vi "KlingerV2 GetStatus.vi"(4 "error in":errorcluster, 7 "VISA Rsrc":refnum<visa-resource-name>="SR530") -> (0 "error out":errorcluster, 1 "Message Cont":string caption="Message de statut", 2 "Statut":bool, 3 "Message D'erreur":string)   [LabVIEW 2019]
doc: "Ce VI effectue une lecture du message de statut du contrôlleur. Celui-ci indique entre autres, si les axes sont en mouvement, la positions de chaque axe, et l'état des interrupteurs de fin de course. De plus, si une erreur c'est produite (ex: commande invalide), il retourrne un code d'erreur avec une brève description. Dans ce dernier cas, le VI rapporte le message d'erreur au VI \"Klinger ErrorHandler\"."
uses:
  <vilib>/Utility/error.llb/DialogType.ctl
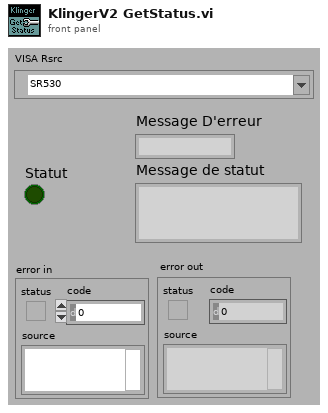
[diagram p1: front panel]
types:
  T1 = enum16{"Lit", "Fin", "Verif erreur", "fixe options", "commande ?"}
  T2 = typedef "DialogType.ctl" = u16
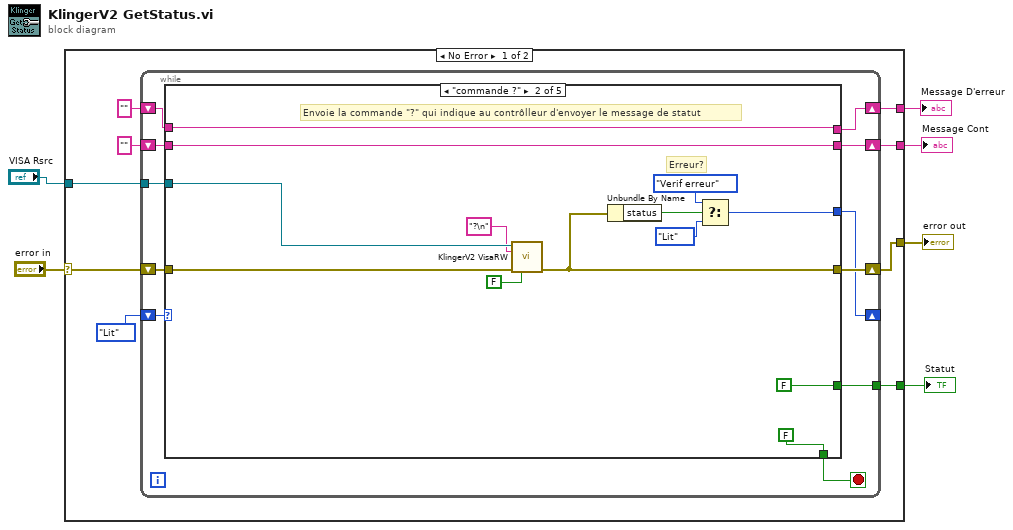
[diagram p0: block diagram]
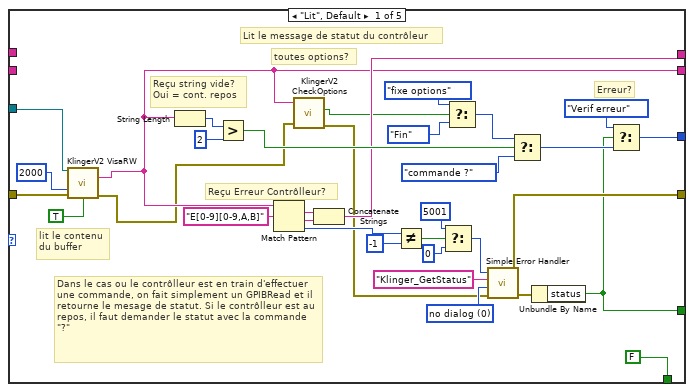
[diagram p2: hidden frame]
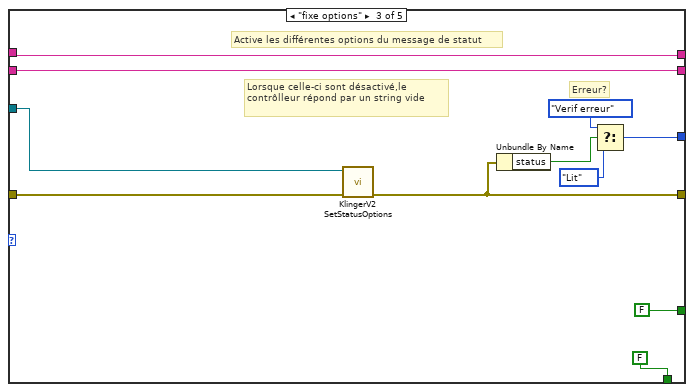
[diagram p3: hidden frame]
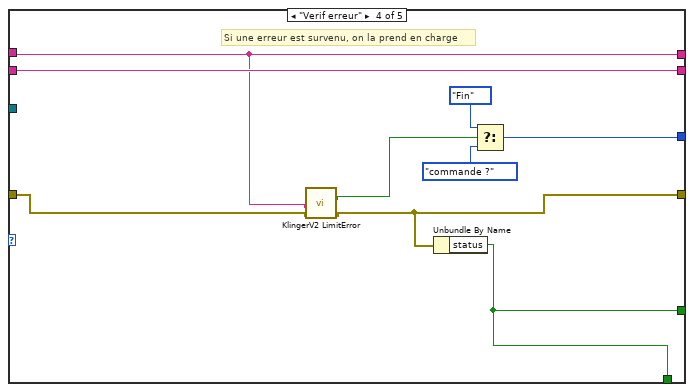
[diagram p4: hidden frame]
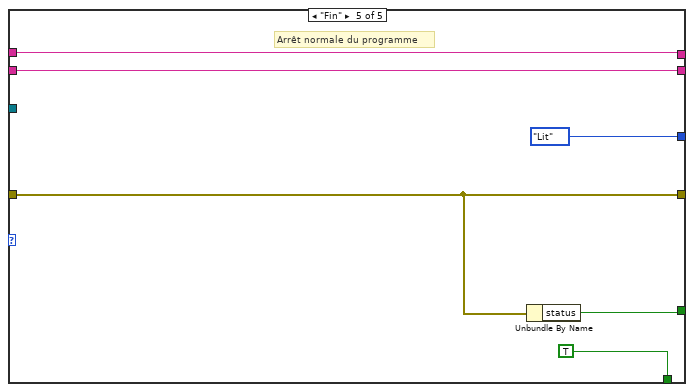
[diagram p5: hidden frame]
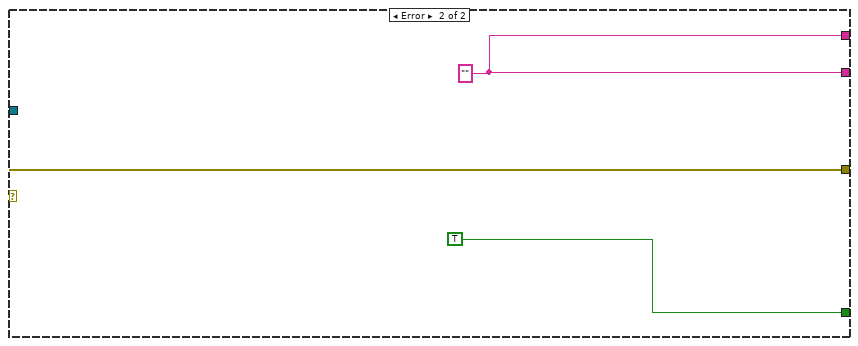
[diagram p6: hidden frame]
diagram:
  n1 = case shown="No Error" "error in" {
    selector: "error in" -> [w15 w101]
    tunnel: [w10 w99] -> w6
    tunnel: [w9 w101] -> w5
    tunnel: [w11 TRUE] -> w4
    tunnel: "VISA Rsrc" -> [w13 _]
    tunnel: [w14 w99] -> w2
    frame No Error {
      n2 = while {
        tunnel: w13 -> [w25]
        tunnel: [w21] -> w11
        shift-right: [w20] -> _
        shift-left: T1."Lit" -> [w24]
        shift-right: [w23] -> w9
        shift-left: w15 -> [w26]
        shift-right: [w22] -> w14
        shift-left: "" ("data") -> [w18]
        shift-right: [w16] -> w10
        shift-left: "" -> [w17]
        stop <- w19 stop-if-true
        n3 = case shown="\"commande ?\"" w24 {
          tunnel: w26 -> [w32 w62 w74 w85 w97]
          tunnel: [w31 w70 w82 w91 w95] -> w22
          tunnel: w25 -> [w30 w64 w75 _ _]
          tunnel: [w40 w61 w73 w86 w97] -> w23
          tunnel: [w39 FALSE FALSE ("status") w88 w98] -> w21
          tunnel: [w43 w65 w76 w92 T1."Lit"] -> w20
          tunnel: [FALSE FALSE FALSE w88 TRUE] -> w19
          tunnel: w18 -> [_ w70 w82 w91 w95]
          tunnel: w17 -> [_ w69 w83 w84 w94]
          tunnel: [w44 w69 w83 w84 w94] -> w16
          frame "Lit", Default {
            w52 = T2 0 items=["no dialog", "OK message", "continue or stop message", "OK message + warnings", "continue/stop + warnings"] ("type of dialog (OK msg:1)")
            # "toutes options?"
            # "Lit le message de statut du contrôleur"
            # "lit le contenu\ndu buffer"
            # "Dans le cas ou le contrôlleur est en train d'effectuer une commande, on fait simplement un GPIBRead et il retourne le mesage de statut. Si le contrôlleur est au repos, il faut demander le statut avec la commande \"?\""
            # "Erreur?"
            # "Reçu string vide?\nOui = cont. repos"
            # "Reçu Erreur Contrôlleur?"
            n4 = call <userlib>:"KlingerV2 VisaRW.vi"("VISA Rsrc"=w30, "Nbcaract"=u32 2000, "error in (no error)"=w32, "Poll?(F)"=TRUE) -> ("ChaineRep"=w31:string, "error out"=w28:errorcluster)  [unwired: 7 in, 3 out]
            n5 = String Length(string=w31) -> (length=w48:i32)
            n6 = Greater?(x=w48, y=2) -> (0:w46:bool)
            n7 = Match Pattern(string=w31, regular expression="E[0-9][0-9,A,B]") -> (match substring=w57:string, after substring=w56:string, offset past match=w58:i32)  [unwired: 1 in, 1 out]
            n8 = call <userlib>:"KlingerV2 CheckOptions.vi"("Message Cont"=w31, "error in"=w28) -> ("Statut"=w35:bool, "error out"=w34:errorcluster)  [unwired: 7 in]
            n9 = Concatenate Strings(w57, w56) -> (w44:string)
            n10 = Not Equal?(x=w58, y=-1) -> (x != y?=w51:bool)
            n11 = Select(t=5001 ("error code (no error:0)"), s=w51, f=0) -> (s? t:f=w53:i32)
            n12 = Select(t=T1."fixe options", s=w35, f=T1."Fin") -> (s? t:f=w38:T1)
            n13 = call <vilib>:"Simple Error Handler.vi"("error code (no error:0)"=w53, "error source (\" \")"="Klinger_GetStatus" ("error source (\" \")"), "type of dialog (OK msg:1)"=w52, "error in (no error)"=w34) -> ("error out"=w40:errorcluster)  [unwired: 1 in, 4 out]
            n14 = Select(t=w38, s=w46, f=T1."commande ?") -> (s? t:f=w42:T1)
            n15 = Unbundle By Name(w40) -> ("status"=w39:bool)
            n16 = Select(t=T1."Verif erreur", s=w39, f=w42) -> (s? t:f=w43:T1)
          }
          frame "commande ?" {
            # "Erreur?"
            # "Envoie la commande \"?\" qui indique au contrôlleur d'envoyer le message de statut"
            n17 = call <userlib>:"KlingerV2 VisaRW.vi"("VISA Rsrc"=w64, "ChaineCom"="?\n" ("data"), "error in (no error)"=w62, "Lecture?(T)"=FALSE) -> ("error out"=w61:errorcluster)  [unwired: 7 in, 4 out]
            n18 = Unbundle By Name(w61) -> ("status"=w68:bool)
            n19 = Select(t=T1."Verif erreur", s=w68, f=T1."Lit") -> (s? t:f=w65:T1)
          }
          frame "fixe options" {
            # "Erreur?"
            # "Lorsque celle-ci sont désactivé,le contrôlleur répond par un string vide"
            # "Active les différentes options du message de statut"
            n20 = call <userlib>:"KlingerV2 SetStatusOptions.vi"("error in"=w74, "VISA Rsrc"=w75) -> ("error out"=w73:errorcluster)  [unwired: 5 in]
            n21 = Unbundle By Name(w73) -> ("status"=w79:bool)
            n22 = Select(t=T1."Verif erreur", s=w79, f=T1."Lit") -> (s? t:f=w76:T1)
          }
          frame "Verif erreur" {
            # "Si une erreur est survenu, on la prend en charge"
            n23 = call <userlib>:"KlingerV2 LimitError.vi"("Message d'erreur"=w84, "Error In"=w85) -> ("Statut"=w87:bool, "Error out"=w86:errorcluster)  [unwired: 5 in]
            n24 = Unbundle By Name(w86) -> ("status"=w88:bool)
            n25 = Select(t=T1."Fin", s=w87, f=T1."commande ?") -> (s? t:f=w92:T1)
          }
          frame "Fin" {
            # "Arrêt normale du programme"
            n26 = Unbundle By Name(w97) -> ("status"=w98:bool)
          }
        }
      }
    }
    frame Error {
      w99 = "" ("data")
    }
  }
  "error out" <- w5
  "Statut" <- w4
  "Message D'erreur" <- w6
  "Message Cont" <- w2
